vi "Host 25042.vi"() -> ()   [LabVIEW 2018]
uses:
  <instrlib>/niDCPower/nidcpower.llb/niDCPower Measurement Type.ctl
panel:
  in  "Пельтье":bool
  in  "Период опроса, мс":u32=1
  in  "Стоп":bool
  in  "Питание":bool
  in  "SEL_T, мс":u32=100
  in  "SIM_SEL":bool
  out "SEL":bool
  in  "0.0_selcur":dbl=0.3 caption="current limit" format="%_6p"
  in  "1.0_selcur":dbl=0.3 caption="current limit" format="%_6p"
  out "0.0":i32
  out "0.0":bool
  out "1.0":i32
  out "1.0":bool
  in  "0.0, V":dbl=5.0 caption="voltage level" format="%_6p"
  in  "0.0_curlim, A":dbl=0.5 caption="current limit" format="%_6p"
  in  "Пельтье_curlim, A":dbl=0.5 caption="current limit" min=0.01 max=2.0 format="%_6p"
  out "0.0_cur, A":dbl caption="measurement" format="%_6g"
  out "Пельтье_cur, A":dbl caption="measurement" format="%_6g"
  in  "Пельтье, V":dbl=5.0 caption="voltage level" min=0.0 max=20.0 format="%_6p"
  in  "1.0, V":dbl=5.0 caption="voltage level" format="%_6p"
  in  "1.0_curlim, A":dbl=0.5 caption="current limit" format="%_6p"
  out "1.0_cur, A":dbl caption="measurement" format="%_6g"
  out "0.1 Chart":dbl(graph)=-0.0025072983641264367
  out "1.0 Chart":dbl(graph)=-0.0403673797130392
  out "0.0 Chart":dbl(graph)=0.17110122624002952 caption="Waveform Chart 5"
  in  "0.0/0.1":refnum<k15>="PXI1Slot2" caption="instrument handle"
  in  "1.0/1.1":refnum<k15>="PXI1Slot3" caption="instrument handle"
  in  "SEL":path=path "C:/Users/agest/Downloads/Telegram Desktop/25_042_ИКИ РАН/SEL"
  out "Номер образца":string="0"
  # "Для ТЗЧ:\n0.0 - питание ПЛИС\n1.0 - питание матрицы\n\n0.1+1.1 - Пельтье"
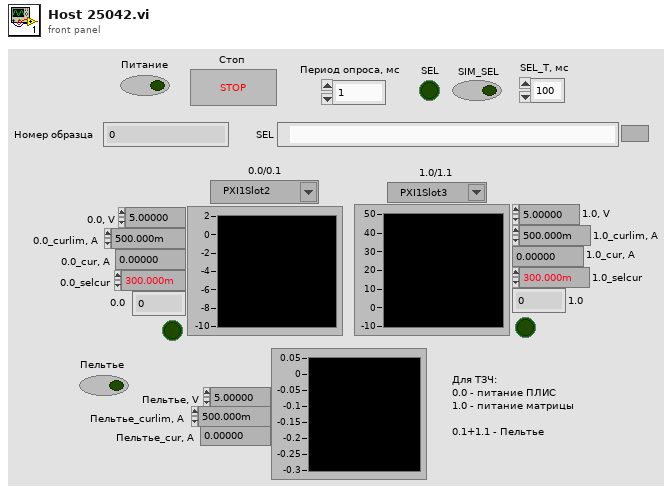
[diagram p1: front panel]
types:
  T1 = enum16{"open", "replace", "create", "open or create", "replace or create", "replace or create with confirmation"}
  T2 = typedef "niDCPower Measurement Type.ctl" = i32
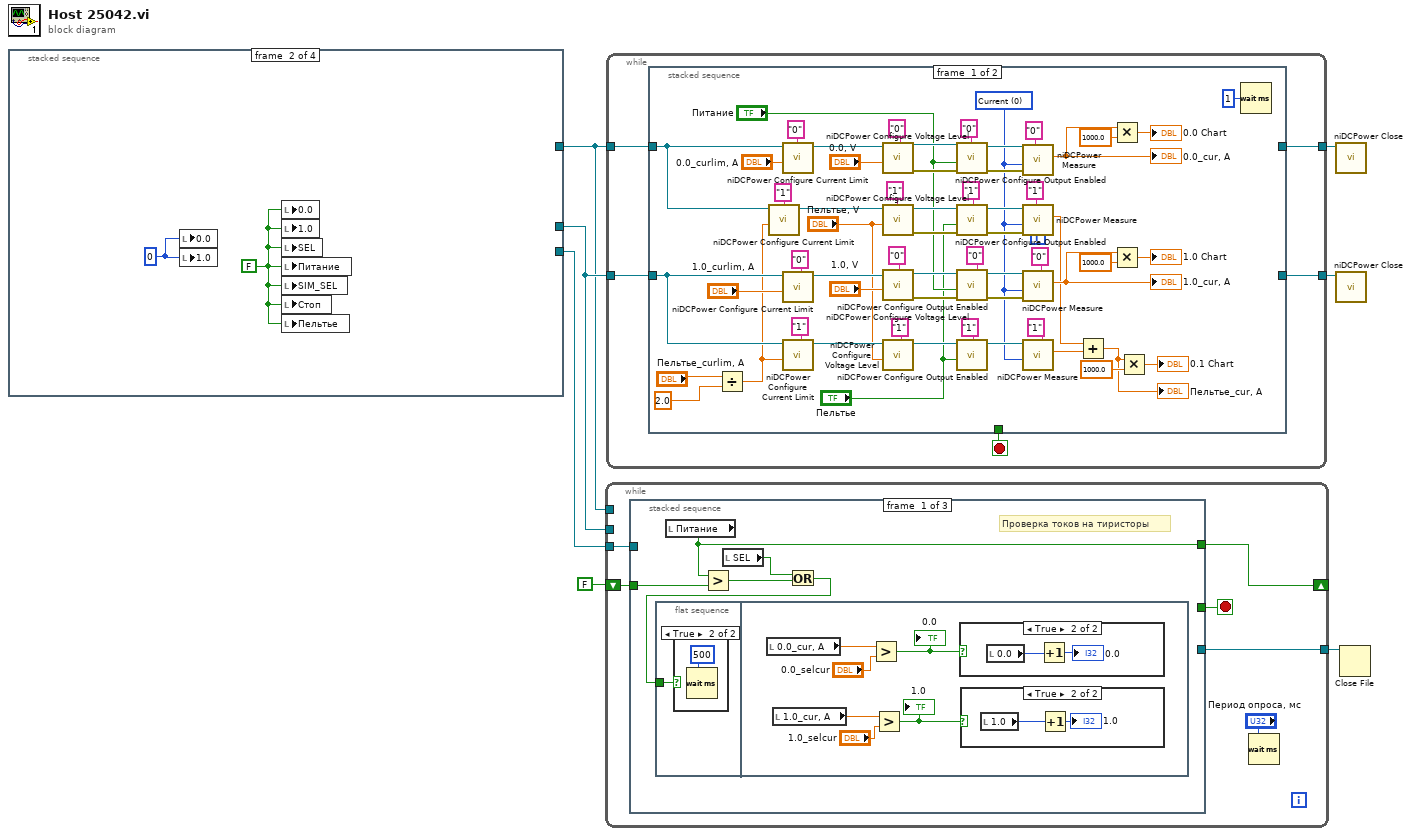
[diagram p0: block diagram]
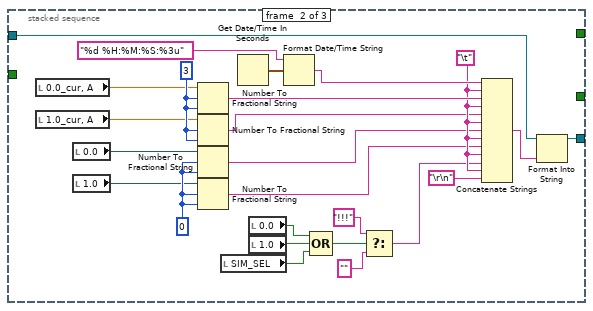
[diagram p5: hidden frame]
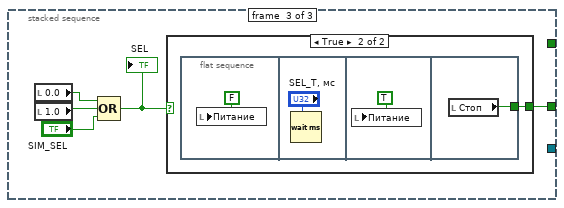
[diagram p6: hidden frame]
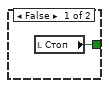
[diagram p7: hidden frame]
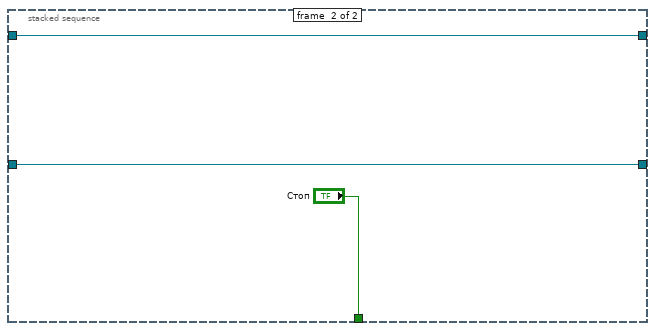
[diagram p8: hidden frame]
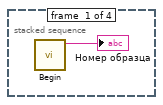
[diagram p9: hidden frame]
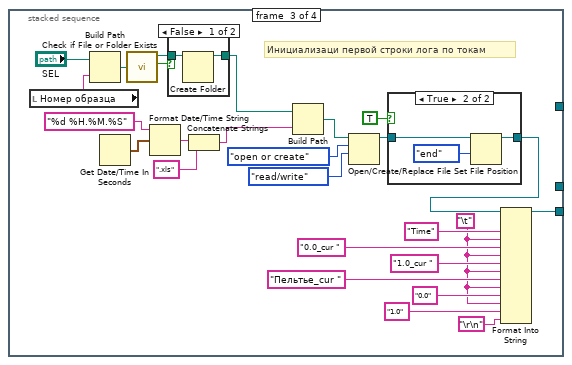
[diagram p10: hidden frame]
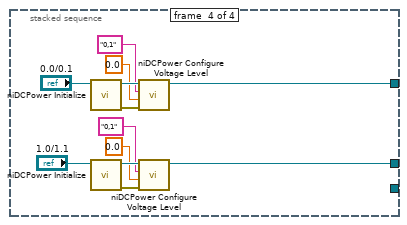
[diagram p13: hidden frame]
diagram:
  n1 = stacked-sequence {
    tunnel: [_ _ _ w45] -> w4
    tunnel: [_ _ _ w44] -> w3
    tunnel: [_ _ w20 _] -> w6
    frame #0 {
      n2 = call "Begin.vi"() -> ("Номер образца 2"=→"Номер образца":string)  [unwired: 11 in]
    }
    frame #1 {
      w10 = 0
      w9 = FALSE
      n3 = local write "0.0"(w10) -> ()
      n4 = local write "1.0"(w10) -> ()
      n5 = local write "0.0"(w9) -> ()
      n6 = local write "1.0"(w9) -> ()
      n7 = local write "SEL"(w9) -> ()
      n8 = local write "Питание"(w9) -> ()
      n9 = local write "SIM_SEL"(w9) -> ()
      n10 = local write "Стоп"(w9) -> ()
      n11 = local write "Пельтье"(w9) -> ()
    }
    frame #2 {
      w13 = "\t"
      # "Инициализаци первой строки лога по токам"
      n12 = local read "Номер образца"() -> (w32:string)
      n13 = Build Path(base path="SEL", name or relative path=w32) -> (appended path=w34:path)
      n14 = Get Date/Time In Seconds() -> (seconds since 1Jan1904=w27:timestamp)
      n15 = call <vilib>:"Check if File or Folder Exists.vi"("path"=w34) -> ("file or folder exists?"=w35:bool, "dup path"=w36:path)  [unwired: 8 in, 1 out]
      n16 = Format Date/Time String(time format string (%c)="%d %H.%M.%S", seconds (now)=w27) -> (date/time string=w24:string)  [unwired: 1 in]
      n17 = case shown="False" w35 {
        tunnel: w36 -> [w42 w43]
        tunnel: [w41 w43] -> w19
        frame False {
          n18 = Create Folder(path (use dialog)=w42) -> (created path=w41:path)  [unwired: 2 in, 2 out]
        }
        frame True {
        }
      }
      n19 = Concatenate Strings(w24, ".xls" ("string")) -> (w22:string)
      n20 = Build Path(base path=w19, name or relative path=w22) -> (appended path=w25:path)
      n21 = Open/Create/Replace File(file path (use dialog)=w25, operation (0:open)=T1."open or create", access (0:read/write)=enum16{"read/write", "read-only", "write-only"}."read/write") -> (refnum out=w28:refnum<file>)  [unwired: 3 in, 2 out]
      n22 = case shown="True" TRUE {
        tunnel: w28 -> [w37 w40]
        tunnel: [w37 w38] -> w21
        frame False {
        }
        frame True {
          n23 = Set File Position(refnum=w40, from (0:start)=enum16{"start", "end", "current"}."end") -> (refnum out=w38:refnum<file>)  [unwired: 2 in, 1 out]
        }
      }
      n24 = Format Into String(initial string=w21, "Time" ("input 1"), w13, "0.0_cur " ("input 1"), w13, "1.0_cur " ("input 1"), w13, "Пельтье_cur " ("input 1"), w13, "0.0" ("input 1"), w13, "1.0" ("input 1"), "\r\n") -> (resulting string=w20:refnum<file>)  [unwired: 2 in, 1 out]
    }
    frame #3 {
      n25 = call <instrlib>:"niDCPower Initialize.vi"("resource name"="0.0/0.1") -> ("error out"=w52:errorcluster, "instrument handle out"=w54:refnum<k15>)  [unwired: 3 in, 6 out]
      n26 = call <instrlib>:"niDCPower Initialize.vi"("resource name"="1.0/1.1") -> ("error out"=w53:errorcluster, "instrument handle out"=w55:refnum<k15>)  [unwired: 3 in, 6 out]
      n27 = call <instrlib>:"niDCPower Configure Voltage Level.vi"("error in (no error)"=w52, "voltage level"=0.0, "channel name"="0,1", "instrument handle"=w54) -> ("instrument handle out"=w44:refnum<k15>)  [unwired: 6 in, 1 out]
      n28 = call <instrlib>:"niDCPower Configure Voltage Level.vi"("error in (no error)"=w53, "voltage level"=0.0, "channel name"="0,1", "instrument handle"=w55) -> ("instrument handle out"=w45:refnum<k15>)  [unwired: 6 in, 1 out]
    }
  }
  n29 = while {
    shift-right: [w61] -> _
    shift-left: FALSE -> [w60]
    tunnel: w6 -> [w59]
    tunnel: [w57] -> w5
    tunnel: w4 -> [_]
    tunnel: w3 -> [_]
    stop <- w58 stop-if-true
    n30 = stacked-sequence {
      tunnel: [w65 _ _] -> w61
      tunnel: w60 -> [w66 _ _]
      tunnel: w59 -> [_ w98 _]
      tunnel: [_ _ w108] -> w58
      tunnel: [_ w97 _] -> w57
      frame #0 {
        # "Проверка токов на тиристоры"
        n31 = flat-sequence {
          tunnel: w62 -> [w67]
          frame #0 {
            n32 = case shown="True" w67 {
              frame False {
              }
              frame True {
                n33 = Wait (ms)(milliseconds to wait=u32 500) -> ()  [unwired: 1 out]
              }
            }
          }
          frame #1 {
            n34 = local read "0.0_cur, A"() -> (w70:dbl)
            n35 = local read "1.0_cur, A"() -> (w69:dbl)
            n36 = Greater?(x=w70, y="0.0_selcur") -> (0:w73:bool)
            "0.0" <- w73
            n37 = Greater?(x=w69, y="1.0_selcur") -> (0:w71:bool)
            "1.0" <- w71
            n38 = case shown="True" w73 {
              frame False {
              }
              frame True {
                n39 = local read "0.0"() -> (w78:i32)
                n40 = Increment(x=w78) -> (x+1=→"0.0":i32)
              }
            }
            n41 = case shown="True" w71 {
              frame False {
              }
              frame True {
                n42 = local read "1.0"() -> (w76:i32)
                n43 = Increment(x=w76) -> (x+1=→"1.0":i32)
              }
            }
          }
        }
        n44 = local read "Питание"() -> (w65:bool)
        n45 = Greater?(x=w65, y=w66) -> (0:w64:bool)
        n46 = local read "SEL"() -> (w63:bool)
        n47 = Or(x=w63, y=w64) -> (x .or. y?=w62:bool)
      }
      frame #1 {
        w95 = i16 0 ("width (-)")
        w96 = i16 3 ("width (-)")
        w84 = "\t"
        n48 = local read "0.0_cur, A"() -> (w94:dbl)
        n49 = local read "1.0_cur, A"() -> (w93:dbl)
        n50 = local read "0.0"() -> (w92:i32)
        n51 = local read "1.0"() -> (w91:i32)
        n52 = Number To Fractional String(number=w94, width (-)=w96, precision (6)=w96) -> (F-format string=w89:string)  [unwired: 1 in]
        n53 = Number To Fractional String(number=w93, width (-)=w96, precision (6)=w96) -> (F-format string=w83:string)  [unwired: 1 in]
        n54 = Number To Fractional String(number=w92, width (-)=w95, precision (6)=w95) -> (F-format string=w82:string)  [unwired: 1 in]
        n55 = Number To Fractional String(number=w91, width (-)=w95, precision (6)=w95) -> (F-format string=w81:string)  [unwired: 1 in]
        n56 = local read "SIM_SEL"() -> (w85:bool)
        n57 = Get Date/Time In Seconds() -> (seconds since 1Jan1904=w103:timestamp)
        n58 = local read "0.0"() -> (w87:bool)
        n59 = local read "1.0"() -> (w86:bool)
        n60 = Format Date/Time String(time format string (%c)="%d %H:%M:%S:%3u", seconds (now)=w103) -> (date/time string=w90:string)  [unwired: 1 in]
        n61 = Compound Arithmetic op=OR(w87, w86, w85) -> (w88:bool)
        n62 = Select(t="!!!", s=w88, f="") -> (s? t:f=w80:string)
        n63 = Concatenate Strings(w90, w84, w89, w84, w83, w84, w82, w84, w81, w84, w80, w84, "\r\n") -> (w102:string)
        n64 = Format Into String(initial string=w98, w102) -> (resulting string=w97:refnum<file>)  [unwired: 2 in, 1 out]
      }
      frame #2 {
        n65 = local read "0.0"() -> (w106:bool)
        n66 = local read "1.0"() -> (w105:bool)
        n67 = Compound Arithmetic op=OR(w106, w105, "SIM_SEL") -> (w107:bool)
        "SEL" <- w107
        n68 = case shown="True" w107 {
          tunnel: [w109 w110] -> w108
          frame False {
            n69 = local read "Стоп"() -> (w109:bool)
          }
          frame True {
            n70 = flat-sequence {
              tunnel: [w114] -> w110
              frame #0 {
                n71 = local write "Питание"(FALSE ("SYS_RESET")) -> ()
              }
              frame #1 {
                n72 = Wait (ms)(milliseconds to wait="SEL_T, мс") -> ()  [unwired: 1 out]
              }
              frame #2 {
                n73 = local write "Питание"(TRUE ("SYS_RESET")) -> ()
              }
              frame #3 {
                n74 = local read "Стоп"() -> (w114:bool)
              }
            }
          }
        }
      }
    }
    n75 = Wait (ms)(milliseconds to wait="Период опроса, мс") -> ()  [unwired: 1 out]
  }
  n76 = while {
    tunnel: w3 -> [w119]
    tunnel: w4 -> [w118]
    tunnel: [w117] -> w2
    tunnel: [w116] -> w1
    stop <- w115 stop-if-true
    n77 = stacked-sequence {
      tunnel: w118 -> [w130 w180]
      tunnel: w119 -> [w129 w181]
      tunnel: [_ w181] -> w117
      tunnel: [_ w180] -> w116
      tunnel: [_ "Стоп"] -> w115
      frame #0 {
        w131 = T2 0 items=["Current", "Voltage"] ("measurement type")
        n78 = Divide(x="Пельтье_curlim, A", y=2.0) -> (x/y=w123:dbl)
        n79 = call <instrlib>:"niDCPower Configure Current Limit.vi"("current limit"=w123, "channel name"="1", "instrument handle"=w129) -> ("instrument handle out"=w170:refnum<k15>)  [unwired: 7 in, 1 out]
        n80 = call <instrlib>:"niDCPower Configure Current Limit.vi"("current limit"="0.0_curlim, A", "channel name"="0", "instrument handle"=w129) -> ("instrument handle out"=w169:refnum<k15>)  [unwired: 7 in, 1 out]
        n81 = call <instrlib>:"niDCPower Configure Current Limit.vi"("current limit"="1.0_curlim, A", "channel name"="0", "instrument handle"=w130) -> ("instrument handle out"=w152:refnum<k15>)  [unwired: 7 in, 1 out]
        n82 = call <instrlib>:"niDCPower Configure Current Limit.vi"("current limit"=w123, "channel name"="1", "instrument handle"=w130) -> ("instrument handle out"=w137:refnum<k15>)  [unwired: 7 in, 1 out]
        n83 = call <instrlib>:"niDCPower Configure Voltage Level.vi"("voltage level"="0.0, V", "channel name"="0", "instrument handle"=w169) -> ("error out"=w162:errorcluster, "instrument handle out"=w165:refnum<k15>)  [unwired: 7 in]
        n84 = call <instrlib>:"niDCPower Configure Voltage Level.vi"("voltage level"="Пельтье, V", "channel name"="1", "instrument handle"=w170) -> ("error out"=w163:errorcluster, "instrument handle out"=w164:refnum<k15>)  [unwired: 7 in]
        n85 = call <instrlib>:"niDCPower Configure Voltage Level.vi"("voltage level"="1.0, V", "channel name"="0", "instrument handle"=w152) -> ("error out"=w156:errorcluster, "instrument handle out"=w157:refnum<k15>)  [unwired: 7 in]
        n86 = call <instrlib>:"niDCPower Configure Voltage Level.vi"("voltage level"="Пельтье, V", "channel name"="1", "instrument handle"=w137) -> ("instrument handle out"=w135:refnum<k15>)  [unwired: 7 in, 1 out]
        n87 = call <instrlib>:"niDCPower Configure Output Enabled.vi"("error in (no error)"=w162, "output enabled"="Питание", "channel name"="0", "instrument handle"=w165) -> ("error out"=w173:errorcluster, "instrument handle out"=w172:refnum<k15>)  [unwired: 6 in]
        n88 = call <instrlib>:"niDCPower Configure Output Enabled.vi"("error in (no error)"=w163, "output enabled"="Пельтье", "channel name"="1", "instrument handle"=w164) -> ("error out"=w174:errorcluster, "instrument handle out"=w175:refnum<k15>)  [unwired: 6 in]
        n89 = call <instrlib>:"niDCPower Configure Output Enabled.vi"("error in (no error)"=w156, "output enabled"="Питание", "channel name"="0", "instrument handle"=w157) -> ("error out"=w148:errorcluster, "instrument handle out"=w149:refnum<k15>)  [unwired: 6 in]
        n90 = call <instrlib>:"niDCPower Configure Output Enabled.vi"("output enabled"="Пельтье", "channel name"="1", "instrument handle"=w135) -> ("instrument handle out"=w133:refnum<k15>)  [unwired: 7 in, 1 out]
        n91 = call <instrlib>:"niDCPower Measure.vi"("error in (no error)"=w173, "measurement type"=w131, "channel name"="0", "instrument handle"=w172) -> ("measurement"=w142:dbl)  [unwired: 5 in, 2 out]
        "0.0_cur, A" <- w142
        n92 = call <instrlib>:"niDCPower Measure.vi"("error in (no error)"=w174, "measurement type"=w131, "channel name"="1", "instrument handle"=w175) -> ("measurement"=w121:dbl)  [unwired: 5 in, 2 out]
        n93 = call <instrlib>:"niDCPower Measure.vi"("error in (no error)"=w148, "measurement type"=w131, "channel name"="0", "instrument handle"=w149) -> ("measurement"=w143:dbl)  [unwired: 5 in, 2 out]
        "1.0_cur, A" <- w143
        n94 = call <instrlib>:"niDCPower Measure.vi"("measurement type"=w131, "channel name"="1", "instrument handle"=w133) -> ("measurement"=w122:dbl)  [unwired: 6 in, 2 out]
        n95 = Add(x=w121, y=w122) -> (x+y=w120:dbl)
        "Пельтье_cur, A" <- w120
        n96 = Multiply(x=w142, y=1000.0) -> (x*y=→"0.0 Chart":dbl)
        n97 = Multiply(x=w143, y=1000.0) -> (x*y=→"1.0 Chart":dbl)
        n98 = Multiply(x=w120, y=1000.0) -> (x*y=→"0.1 Chart":dbl)
        n99 = Wait (ms)(milliseconds to wait=u32 1) -> ()  [unwired: 1 out]
      }
      frame #1 {
      }
    }
  }
  n100 = call <instrlib>:"niDCPower Close.vi"("instrument handle"=w2) -> ()  [unwired: 10 in, 1 out]
  n101 = call <instrlib>:"niDCPower Close.vi"("instrument handle"=w1) -> ()  [unwired: 10 in, 1 out]
  n102 = Close File(refnum=w5) -> ()  [unwired: 1 in, 2 out]
